vi "SpeedDistanceM2.vi"(0 "VISA Refnum in":refnum<visa-resource-name>, 1 "Distance":u32 max=127 step=1, 2 "Speed":i32 max=127 step=1, 3 "Address":u8, 5 "error in (no error)":errorcluster) -> (6 "VISA Refnum out":refnum<visa-resource-name>, 7 "Valid":bool, 8 "error out":errorcluster)   [LabVIEW 2015, in "Ion Motion Roboclaw.lvlib"]
uses:
  <instrlib>/Ion Motion Roboclaw/Ion Motion Roboclaw.lvlib
panel:
  in  "Immediate":u8 max=127 step=1
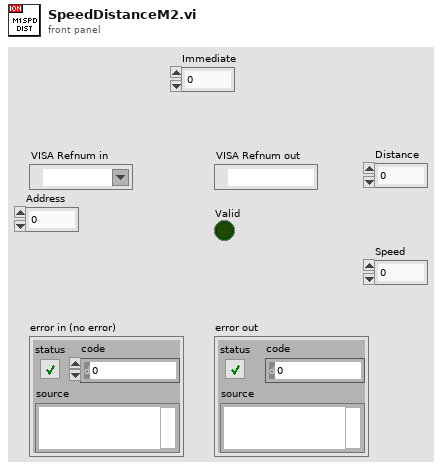
[diagram p1: front panel]
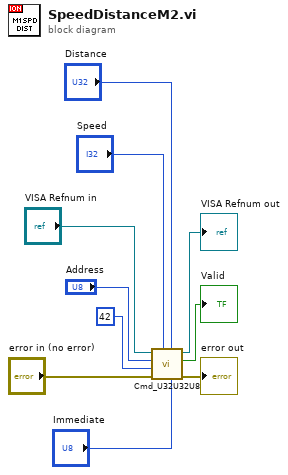
[diagram p0: block diagram]
diagram:
  n1 = call <instrlib>:"Cmd_U32U32U8.vi"("Arg3"="Immediate", "Arg2"="Distance", "Arg1"="Speed", "error in (no error)"="error in (no error)", "Cmd"=u8 42, "Address"="Address", "VISA Refnum in"="VISA Refnum in") -> ("error out"=→"error out":errorcluster, "Valid"=→"Valid":bool, "VISA Refnum out"=→"VISA Refnum out":refnum<visa-resource-name>)  [unwired: 2 in]
